vi "SVD Dispose.vi"(8 "error in (no error)":errorcluster, 11 "SVD in":refnum<class "SVD.lvclass">) -> (0 "error out":errorcluster)   [LabVIEW 2020, in "OpenLvVision_OpenCv.lvlib" / "SVD.lvclass"]
doc: "Closes the reference and triggers cleanup of the associated C++ object, releasing system resources.\nYou must call this VI when you are finished using the object reference to prevent memory leaks!"
uses:
  SVD.lvclass
  C:/Users/lukas/Downloads/OpenLvVision_OpenCv/SourceCode/LabView/OpenLvVision_OpenCv/_LvHelpers/EdvrObject/EdvrObject.lvclass
  _LvHelpers/EdvrObject/EdvrObject.lvclass/EdvrObject.ctl
  _LvHelpers/EdvrObject/EdvrObject.lvclass
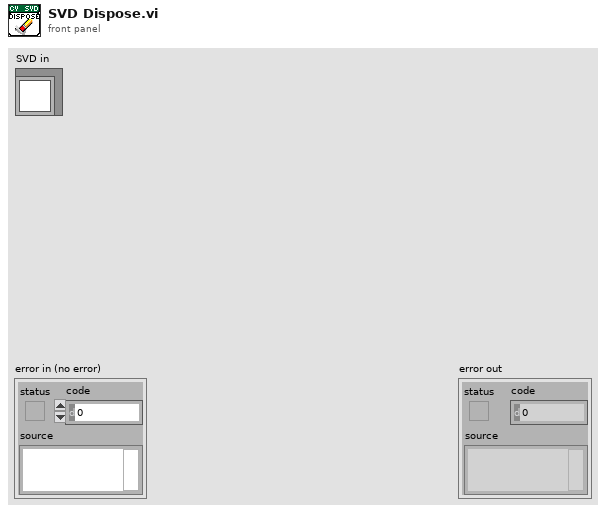
[diagram p1: front panel]
types:
  T1 = typedef "OpenLvVision_OpenCv.lvlib/EdvrObject.lvclass/Edvr.ctl" = refnum<data-value>
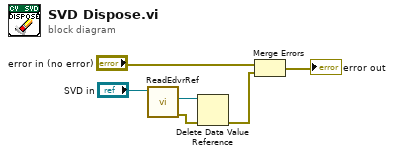
[diagram p0: block diagram]
diagram:
  n1 = call "ReadEdvrRef.vi"("EdvrObject in"="SVD in") -> ("error out"=w5:errorcluster, "Edvr"=w6:T1)  [unwired: 8 in, 1 out]
  n2 = Delete Data Value Reference(data value reference=w6, error in=w5) -> (error out=w4:errorcluster)  [unwired: 1 out]
  n3 = Merge Errors("error in (no error)", w4) -> (→"error out":errorcluster)
